vi "Scan_ConstantDistance.vi"() -> ()   [LabVIEW 2023]
uses:
  Sub_Vi/TypeDefsControls/Iterator.ctl
  Sub_Vi/TypeDefsControls/Xposition.ctl
  Sub_Vi/TypeDefsControls/Yposition.ctl
  Sub_Vi/TypeDefsControls/Piezo Velocity.ctl
  Sub_Vi/TypeDefsControls/Voltage.ctl
  Sub_Vi/TypeDefsControls/Zposition.ctl
  Sub_Vi/TypeDefs/Settings.ctl
  Sub_Vi/TypeDefs/ChangeOnFly.ctl
  Sub_Vi/TypeDefs/Display.ctl
  Sub_Vi/TypeDefsControls/Feedback Type.ctl
  Settings.vi
panel:
  in  "Feedback Type":T1
  in  "Pixels per Line":T2=100.0 min=1.0
  out "Estimated time (mins)":dbl
  in  "Start scan Button":bool
  in  "Retract after \nscan complete":bool=TRUE
  in  "Display Cluster":T3
  in  "ChangeonFly":T4
  in  "SettingsCluster":T5={"Sample Rate (us)"=1, "Samples Per Data Point (int, power of 2)"=1000, "DistanceToBulk (um)"=-1.0, "HoldTimeScaler"=1, "SaveData"=FALSE, "DistanceToBulk (um) 2"=-1.0, "DistanceToBulk (um) 3"=-1.0}
  in  "Greater Than":bool=TRUE
  in  "End Extension (µm)":T6=38.0 min=0.0 max=100000.0
  in  "Pause At End\nOf Line Time (s)":dbl=0.002 min=0.0 max=100.0
  in  "Upper dZ \nlimit  (nm)":i32=8 min=0
  in  "Feedback Threshold (A)":dbl=1e-13
  in  "P":fxp<+/-,32,1>=0.029999999795109034 format="%.32g"
  in  "X Center (µm)":T7=150.0 min=0.0 max=100000.0
  in  "Y Center (µm)":T8=150.0 min=0.0 max=100000.0
  in  "Y Width (µm)":T8=10.0 min=0.0 max=100000.0
  in  "X Width (µm)":T7=10.0 min=0.0 max=100000.0
  in  "Number of Lines":T2=10.0 min=1.0
  in  "Lateral Scan Rate (µm/s)":T9=1.0 min=0.0
  in  "Reverse Scan Voltage (V)":T10=1.0 min=-10.0 max=10.0
  in  "Forward Scan Voltage (V)":T10=1.0 min=-10.0 max=10.0
  in  "Approach Rate (µm/s)":T9=1.0 min=0.0
  in  "Start Extention (µm)":T6 min=0.0 max=100000.0
  in  "Stop":bool
  in  "Pause":bool
  in  "Update Position Loop \nWait Time (ms)":u32=50 min=1 max=32000
  in  "Start Scanning Button":bool
  out "Y end":dbl
  out "X end":dbl
  out "X start":dbl
  out "Y start":dbl
  in  "Tab Control 4":T11(tab)=enum."AC Approach"
  out "Forward Scan Topography":dbl[][](graph)
  out "Reverse Scan Topography":dbl[][](graph)
  out "C1 Forward Scan":dbl[][](graph)
  out "C1 Reverse Scan":dbl[][](graph)
  out "C2 Forward Scan":dbl[][](graph)
  out "C2 Reverse Scan":dbl[][](graph)
  out "t vs Phase":dbl[](graph)
  out "t vs Amp":dbl[](graph)
  out "Z vs C1":cluster{"Y":dbl[], "Y":dbl[]}[](graph)
  out "t vs C2":dbl[](graph)
  out "t vs C1":dbl[](graph)
  # "Approach Settings"
  # "Pause at"
  # "Scan Settings"
  # "Define Scan Area"
  # "Scan Feedback Parameters"
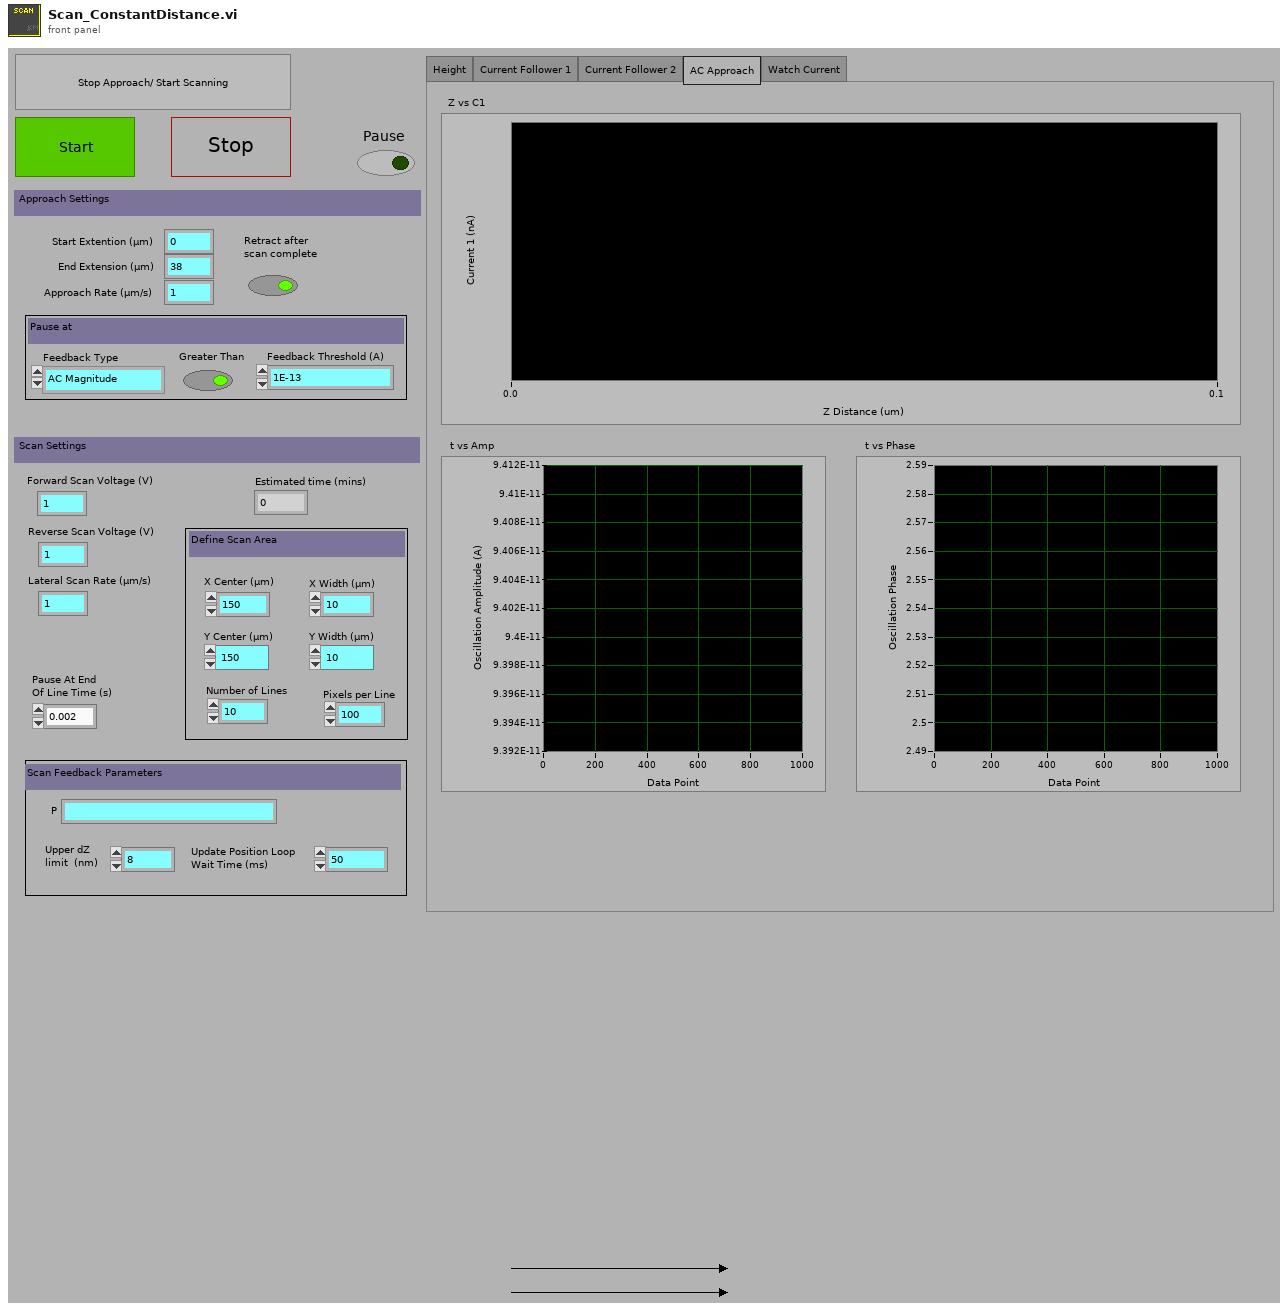
[diagram p1: front panel]
types:
  T1 = typedef "Feedback Type.ctl" = enum16{"AC Magnitude", "Current 1", "Current 2", "Phase"}
  T2 = typedef "Iterator.ctl" = dbl
  T3 = typedef "Display.ctl" = cluster{"X":refnum<vi>, "Y":refnum<vi>, "Z":refnum<vi>, "Amp":refnum<vi>, "Phase":refnum<vi>, "t vs Z":refnum<vi>, "t vs C1":refnum<vi>, "t vs C2":refnum<vi>, "t vs C3":refnum<vi>, "t vs Amp":refnum<vi>, "t vs Phase":refnum<vi>, "t vs X":refnum<vi>, "t vs Y":refnum<vi>, "Z vs C1":refnum<vi>, "Z vs C2":refnum<vi>, "Z vs C3":refnum<vi>, "V vs C1":refnum<vi>, "V vs C2":refnum<vi>, "V vs C3":refnum<vi>, "X/Y/Z F":refnum<vi>, "X/Y/Z R":refnum<vi>, "X/Y/C1 F":refnum<vi>, "X/Y/C1 R":refnum<vi>, "X/Y/C2 F":refnum<vi>, "X/Y/C2 R":refnum<vi>, "X/Y/C3 F":refnum<vi>, "X/Y/C3 R":refnum<vi>, "NumberOfLines":u16, "um Per Pixel":dbl, "um Per Line":dbl, "X Center":dbl, "Hop X/Y/Z":refnum<vi>, "Hop X/Y/C1":refnum<vi>, "Hop X/Y/C2":refnum<vi>, "Hop X/Y/C3":refnum<vi>, "X Width":dbl, "Y Width":dbl, "Hopping Distance":dbl, "V2 vs C1":refnum<vi>, "V vs Phase":refnum<vi>, "Y Center":dbl, "Number of Pixels":dbl, "V2 vs C2":refnum<vi>, "V2 vs C3":refnum<vi>, "V vs y":refnum<vi>, "V2 vs y":refnum<vi>, "Z vs Amp":refnum<vi>, "Z vs Phase":refnum<vi>}
  T4 = typedef "ChangeOnFly.ctl" = cluster{"Stop (boolean)":refnum<vi>, "Pause (boolean)":refnum<vi>, "EndCurrentLine (boolean)":refnum<vi>, "max movement per update step (Interger, nm)":refnum<vi>, "P (float, arb)":refnum<vi>, "Feedback set point (double, Amps)":refnum<vi>, "Voltage (double, V)":refnum<vi>, "Feedback set point 2 (double, Amps)":refnum<vi>, "Stop on Greater Than 2? (boolean)":refnum<vi>, "Stop on Greater Than? (boolean)":refnum<vi>, "Voltage 2 (double, V)":refnum<vi>, "Feedback Type (enum)":refnum<vi>, "Feedback Type 2 (enum)":refnum<vi>}
  T5 = typedef "Settings.ctl" = cluster{"Sample Rate (us)":u32, "Samples Per Data Point (int, power of 2)":i16, "DistanceToBulk (um)":dbl, "HoldTimeScaler":u64, "SaveData":bool, "DistanceToBulk (um) 2":dbl, "DistanceToBulk (um) 3":dbl}
  T6 = typedef "Zposition.ctl" = dbl
  T7 = typedef "Xposition.ctl" = dbl
  T8 = typedef "Yposition.ctl" = dbl
  T9 = typedef "Piezo Velocity.ctl" = dbl
  T10 = typedef "Voltage.ctl" = dbl
  T11 = enum32{"Height", "Current Follower 1", "Current Follower 2", "AC Approach", "Watch Current"}
  T12 = cluster{"Scan Rate (um/s)":dbl, "X Start":dbl, "X End":dbl, "Y Start":dbl, "Y End":dbl, " Z Start":dbl, "Number of Lines":u32, "V":dbl, "Z End":dbl, "Approach Rate (um/s)":dbl, "Squish Approach Rate (um/s)":dbl, "V 2":dbl, "HoldTime / Ticks":u32}
  T13 = typedef "WayPointCluster.ctl" = cluster{"X (um)":dbl[], "Y (um)":dbl[], "Z (um)":dbl[], "V (V)":dbl[], "X Velocity (um s-1)":dbl[], "Y Velocity (um s-1)":dbl[], "Z Velocity (um s-1)":dbl[], "V Velocity (V s-1)":dbl[], "FeedBack Type (enum)":u16[], "Move X (boolean)":bool[], "Move Y (boolean)":bool[], "Move Z (boolean)":bool[], "Move V (boolean)":bool[], "Jump V (boolean)":bool[], "Hold (boolean)":bool[], "Hold Time":u32[], "V2 (V)":dbl[], "Move V2":bool[], "V2 Velocity (V s-1)":dbl[], "Jump V2 (boolean)":bool[], "Update z Position delta (ms)":i16[], "Hold Feedback1":bool[], "Move Z PicoMotor":bool[], " Z PicoMotor Direction":bool[], "DIO0":bool[]}
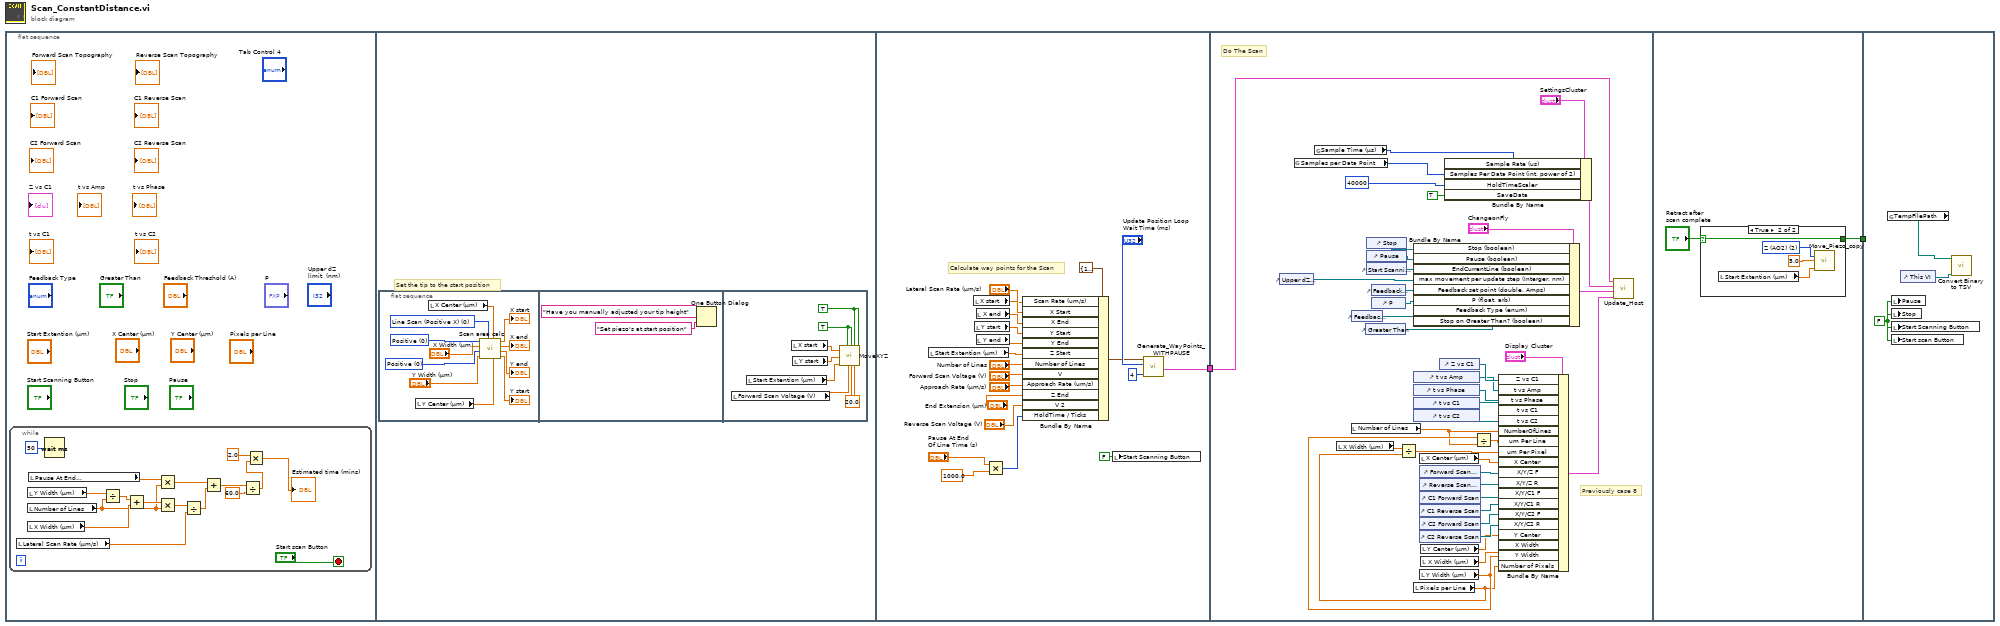
[diagram p0: block diagram]
diagram:
  n1 = flat-sequence {
    tunnel: [w59] -> w2
    tunnel: w2 -> [w71]
    tunnel: [w99] -> w1
    tunnel: w1 -> [_]
    frame #0 {
      n2 = while {
        stop <- "Start scan Button" stop-if-true
        n3 = local read "Lateral Scan Rate (µm/s)"() -> (w15:T9)
        n4 = local read "Number of Lines"() -> (w10:T2)
        n5 = local read "X Width (µm)"() -> (w16:T7)
        n6 = local read "Y Width (µm)"() -> (w18:T8)
        n7 = local read "Pause At End\nOf Line Time (s)"() -> (w13:dbl)
        n8 = Wait (ms)(milliseconds to wait=u32 50) -> ()  [unwired: 1 out]
        n9 = Divide(x=w18, y=w10) -> (x/y=w17:T8)
        n10 = Add(x=w17, y=w16) -> (x+y=w11:T8)
        n11 = Multiply(x=w13, y=w10) -> (x*y=w12:T2)
        n12 = Multiply(x=w11, y=w10) -> (x*y=w9:T8)
        n13 = Divide(x=w9, y=w15) -> (x/y=w14:T8)
        n14 = Add(x=w12, y=w14) -> (x+y=w7:T2)
        n15 = Divide(x=w7, y=60.0) -> (x/y=w4:T2)
        n16 = Multiply(x=2.0, y=w4) -> (x*y=→"Estimated time (mins)":T2)
      }
    }
    frame #1 {
      # "Set the tip to the start position"
      n17 = flat-sequence {
        frame #0 {
          w28 = u16 0 items=["Positive", "Negative"] ("Major Axis Direction")
          w27 = u16 0 items=["Positive", "Negative"] ("Minor Axis Direction")
          w20 = u16 0 items=["Line Scan (Positive X)", "Line Scan (Negative X)", "Line Scan (Positive Y)", "Line Scan (Negative Y)"] ("Scan Type")
          n18 = local read "Y Center (µm)"() -> (w21:T8)
          n19 = local read "X Center (µm)"() -> (w22:T7)
          n20 = call "Scan area calc.vi"("Y Width"="Y Width (µm)", "Major Axis Direction"=w28, "X Width"="X Width (µm)", "Minor Axis Direction"=w27, "Scan Type"=w20, "Y Center"=w21, "X Center"=w22) -> ("Y start"=→"Y start":dbl, "Y end"=→"Y end":dbl, "X end"=→"X end":dbl, "X start"=→"X start":dbl)
        }
        frame #1 {
          n21 = One Button Dialog(message="Have you manually adjusted your tip height", button name ("OK")="Set piezo's at start position") -> ()  [unwired: 1 out]
        }
        frame #2 {
          w35 = TRUE ("Set Z")
          w36 = TRUE ("Set X")
          w37 = 20.0 ("Scan Rate (V/s)")
          n22 = local read "Forward Scan Voltage (V)"() -> (w33:T10)
          n23 = local read "Start Extention (µm)"() -> (w34:T6)
          n24 = local read "X start"() -> (w39:dbl)
          n25 = local read "Y start"() -> (w38:dbl)
          n26 = call "MoveXYZ.vi"("X final height"=w39, "Y final height"=w38, "Z final height"=w34, "Set X"=w36, "V final"=w33, "Set Y"=w36, "Scan Rate (um/s)"=w37, "Set Z"=w35, "Scan Rate (V/s) 2"=w37, "Set Voltage"=w35) -> ()  [unwired: 10 in]
        }
      }
    }
    frame #2 {
      # "Calculate way points for the Scan"
      n27 = local read "Start Extention (µm)"() -> (w45:T6)
      n28 = local read "X start"() -> (w41:dbl)
      n29 = local read "Y start"() -> (w43:dbl)
      n30 = local read "X end"() -> (w42:dbl)
      n31 = local read "Y end"() -> (w44:dbl)
      n32 = Multiply(x="Pause At End\nOf Line Time (s)", y=1000.0) -> (x*y=w54:i64)
      n33 = Bundle By Name(cluster=T12 {"Scan Rate (um/s)"=15.0, "X Start"=15.0, "X End"=15.0, "Y Start"=15.0, "Y End"=15.0, " Z Start"=15.0, "Number of Lines"=15, "V"=15.0, "Z End"=15.0, "Approach Rate (um/s)"=15.0, "Squish Approach Rate (um/s)"=15.0, "V 2"=15.0, "HoldTime / Ticks"=15} ("Input Cluster"), "Scan Rate (um/s)"="Lateral Scan Rate (µm/s)", "X Start"=w41, "X End"=w42, "Y Start"=w43, "Y End"=w44, "Z Start"=w45, "Number of Lines"="Number of Lines", "V"="Forward Scan Voltage (V)", "Approach Rate (um/s)"="Approach Rate (µm/s)", "Z End"="End Extension (µm)", "V 2"="Reverse Scan Voltage (V)", "HoldTime / Ticks"=w54) -> (w50:T12)
      n34 = local write "Start Scanning Button"(FALSE ("Start Scanning Button")) -> ()
      n35 = call "Generate_WayPoints_WITHPAUSE.vi"("Update Position Loop Wait Time (ms)"="Update Position Loop \nWait Time (ms)", "Feedback Enum"=u16 4, "Input Cluster"=w50) -> ("output cluster"=w59:T13)  [unwired: 8 in]
    }
    frame #3 {
      # "Previously case 8"
      # "Do The Scan"
      n36 = control-ref of="Upper dZ \nlimit  (nm)"() -> (w94:refnum<vi>)
      n37 = global read "Settings.vi" "Samples per Data Point"() -> (w72:u16)
      n38 = global read "Settings.vi" "Sample Time (µs)"() -> (w73:u32)
      n39 = local read "X Width (µm)"() -> (w90:T7)
      n40 = local read "Number of Lines"() -> (w76:T2)
      n41 = control-ref of="Feedback Type"() -> (w74:refnum<vi>)
      n42 = control-ref of="Greater Than"() -> (w68:refnum<vi>)
      n43 = control-ref of="Stop"() -> (w92:refnum<vi>)
      n44 = control-ref of="Pause"() -> (w93:refnum<vi>)
      n45 = control-ref of="Start Scanning Button"() -> (w95:refnum<vi>)
      n46 = control-ref of="Feedback Threshold (A)"() -> (w70:refnum<vi>)
      n47 = control-ref of="P"() -> (w69:refnum<vi>)
      n48 = control-ref of="t vs Amp"() -> (w62:refnum<vi>)
      n49 = control-ref of="t vs Phase"() -> (w64:refnum<vi>)
      n50 = control-ref of="t vs C1"() -> (w91:refnum<vi>)
      n51 = control-ref of="t vs C2"() -> (w65:refnum<vi>)
      n52 = local read "Pixels per Line"() -> (w66:T2)
      n53 = Divide(x=w90, y=w66) -> (x/y=w89:T7)
      n54 = Bundle By Name(cluster="ChangeonFly", "Stop (boolean)"=w92, "Pause (boolean)"=w93, "EndCurrentLine (boolean)"=w95, "max movement per update step (Interger, nm)"=w94, "Feedback set point (double, Amps)"=w70, "P (float, arb)"=w69, "Feedback Type (enum)"=w74, "Stop on Greater Than? (boolean)"=w68) -> (w96:T4)
      n55 = control-ref of="Forward Scan Topography"() -> (w88:refnum<vi>)
      n56 = control-ref of="Reverse Scan Topography"() -> (w87:refnum<vi>)
      n57 = control-ref of="C1 Forward Scan"() -> (w86:refnum<vi>)
      n58 = control-ref of="C1 Reverse Scan"() -> (w85:refnum<vi>)
      n59 = control-ref of="C2 Forward Scan"() -> (w84:refnum<vi>)
      n60 = control-ref of="C2 Reverse Scan"() -> (w83:refnum<vi>)
      n61 = local read "X Center (µm)"() -> (w67:T7)
      n62 = local read "Y Width (µm)"() -> (w77:T8)
      n63 = local read "Y Center (µm)"() -> (w79:T8)
      n64 = local read "X Width (µm)"() -> (w78:T7)
      n65 = control-ref of="Z vs C1"() -> (w63:refnum<vi>)
      n66 = Bundle By Name(cluster="SettingsCluster", "Sample Rate (us)"=w73, "Samples Per Data Point (int, power of 2)"=w72, "HoldTimeScaler"=u64 40000, "SaveData"=TRUE) -> (w97:T5)
      n67 = Divide(x=w77, y=w76) -> (x/y=w75:T8)
      n68 = Bundle By Name(cluster="Display Cluster", "Z vs C1"=w63, "t vs Amp"=w62, "t vs Phase"=w64, "t vs C1"=w91, "t vs C2"=w65, "NumberOfLines"=w76, "um Per Line"=w75, "um Per Pixel"=w89, "X Center"=w67, "X/Y/Z F"=w88, "X/Y/Z R"=w87, "X/Y/C1 F"=w86, "X/Y/C1 R"=w85, "X/Y/C2 F"=w84, "X/Y/C2 R"=w83, "Y Center"=w79, "X Width"=w78, "Y Width"=w77, "Number of Pixels"=w66) -> (w98:T3)
      n69 = call "Update_Host.vi"("Display Cluster"=w98, "ChangeonFly"=w96, "SettingsCluster"=w97, "WayPointCluster"=w71) -> ()  [unwired: 6 in]
    }
    frame #4 {
      n70 = case shown="True" "Retract after \nscan complete" {
        selector: "Retract after \nscan complete" -> [w101 w102]
        tunnel: [w101 w102] -> w99
        frame False {
        }
        frame True {
          w105 = u16 2 items=["X (AO0)", "Y (AO1)", "Z (AO2)", "V (AO3)"] ("Channel")
          n71 = local read "Start Extention (µm)"() -> (w103:T6)
          n72 = call "Move_Piezo_copy.vi"("Piezo"=w105, "Movement Speed (µm/s)"=5.0 ("Scan Rate (um/s)"), "Position (µm) (or V)"=w103) -> ()  [unwired: 13 in]
        }
      }
    }
    frame #5 {
      w107 = FALSE ("Stop")
      n73 = global read "Settings.vi" "TempFilePath"() -> (w106:path)
      n74 = local write "Pause"(w107) -> ()
      n75 = local write "Stop"(w107) -> ()
      n76 = local write "Start Scanning Button"(w107) -> ()
      n77 = local write "Start scan Button"(w107) -> ()
      n78 = control-ref of="This VI"() -> (w108:refnum<vi>)
      n79 = call "Convert Binary to TSV.vi"("This VI"=w108, "TDMS DataFile Name"=w106) -> ()  [unwired: 10 in]
    }
  }
